vi "Receiver UI.vi"(11 "Error In":errorcluster) -> (15 "Error Out":errorcluster)   [LabVIEW 2022 SP3, in "Receiver.lvclass"]
doc: "This VI acts as a receiver and displays the data received to user."
uses:
  Receiver.lvclass
  Controls/Operation.ctl
  Controls/State Cluster.ctl
  Controls/User Event Operation.ctl
  Controls/Receiver Data Cluster.ctl
  Downloads/Sample PC Template/Sample PC Template/Typedefs/Data.ctl
  Downloads/Sample PC Template/Sample PC Template/Sample PC Template.lvlib
  Data/Data.lvclass
panel:
  out "Receiver Notified":bool
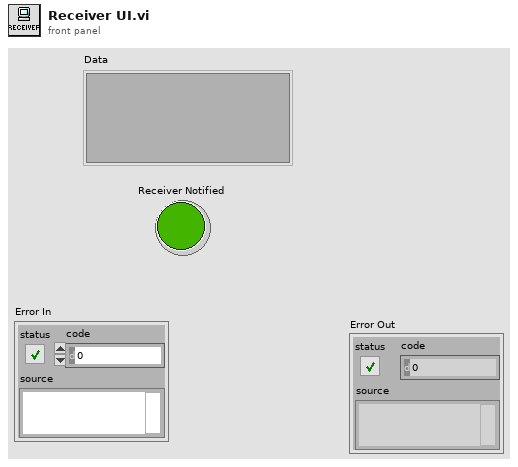
[diagram p1: front panel]
types:
  T1 = typedef "User Event Operation.ctl" = enum16{"Obtain", "Generate", "Release"}
  T2 = typedef "Receiver Data Cluster.ctl" = cluster{"Data":variant, "Receiver UI Triggered":bool, "Data.lvclass":refnum<class "Data.lvclass">, "VI Refnum":refnum<vi>}
  T3 = typedef "State Cluster.ctl" = cluster{"State":string, "Data":variant}
  T4 = typedef "Operation.ctl" = enum16{"Create", "Enqueue", "Enqueue N", "Enstack", "Dequeue", "Flush", "Release"}
  T5 = typedef "Sample PC Template.lvlib/Data.ctl" = cluster{"State":string, "Data":variant}
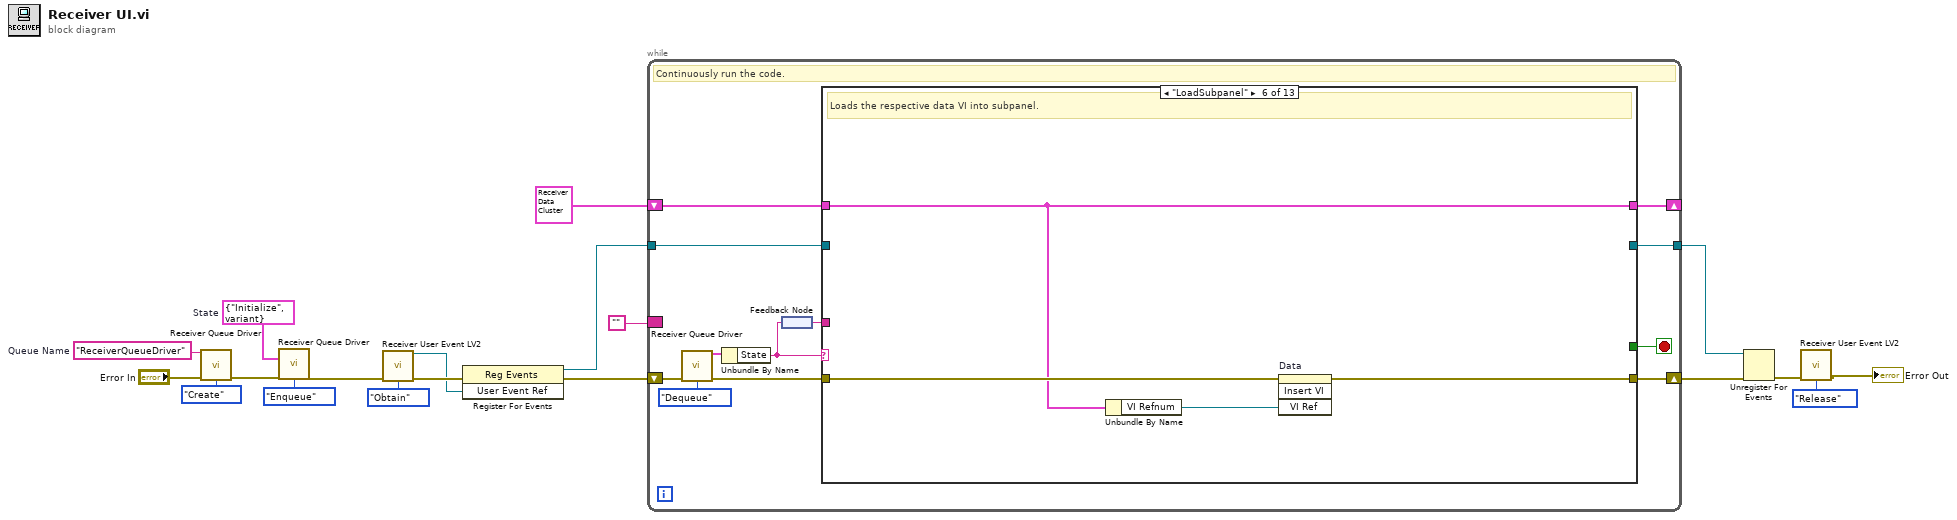
[diagram p0: block diagram]
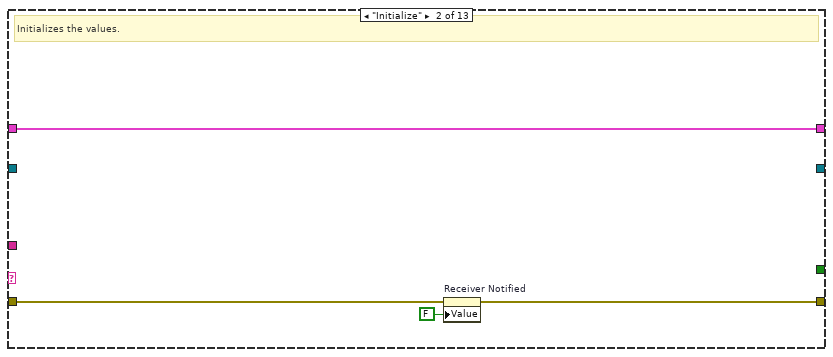
[diagram p3: hidden frame]
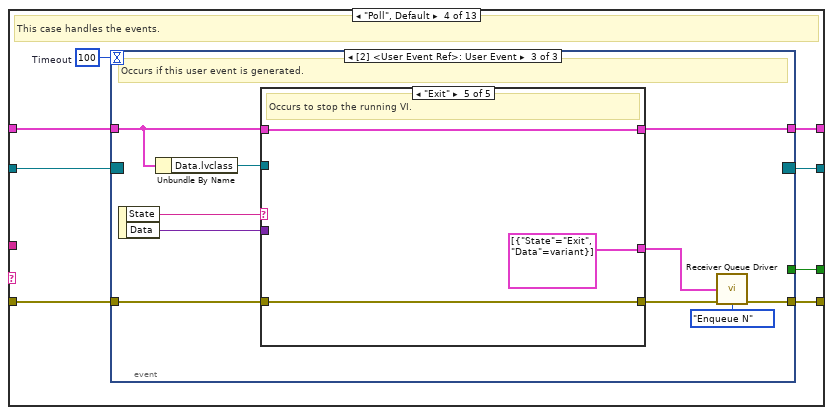
[diagram p5: hidden frame]
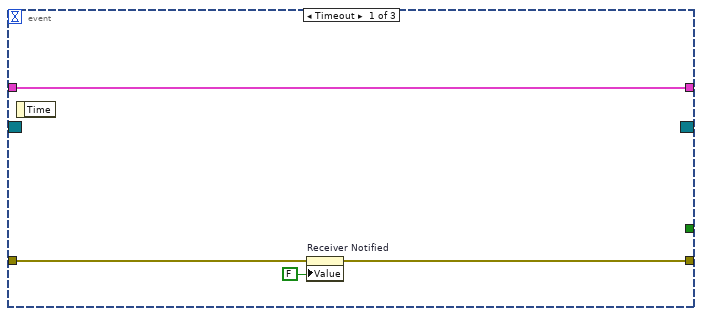
[diagram p6: hidden frame]
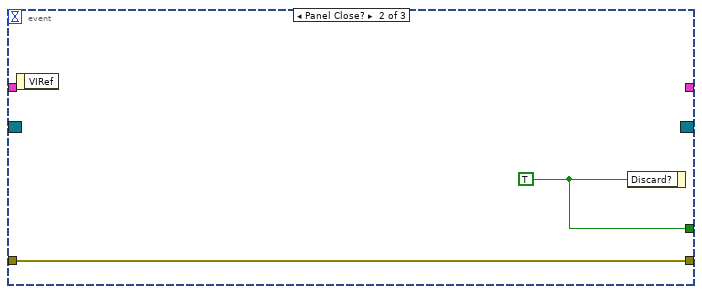
[diagram p7: hidden frame]
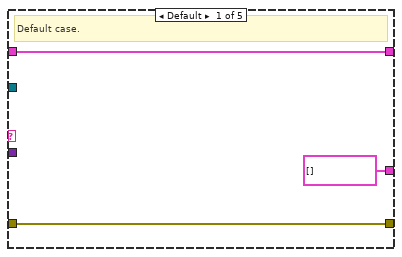
[diagram p8: hidden frame]
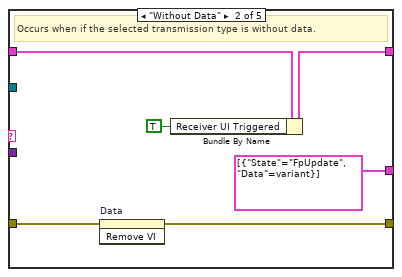
[diagram p9: hidden frame]
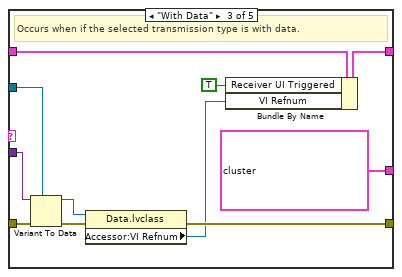
[diagram p10: hidden frame]
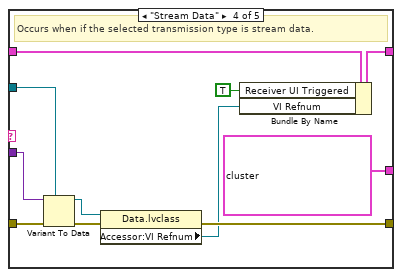
[diagram p11: hidden frame]
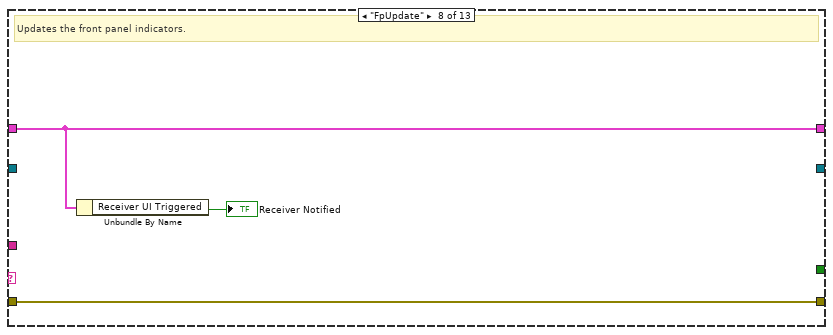
[diagram p14: hidden frame]
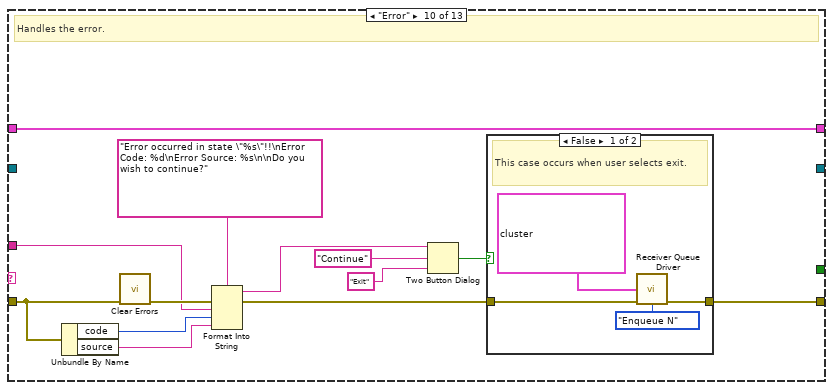
[diagram p16: hidden frame]
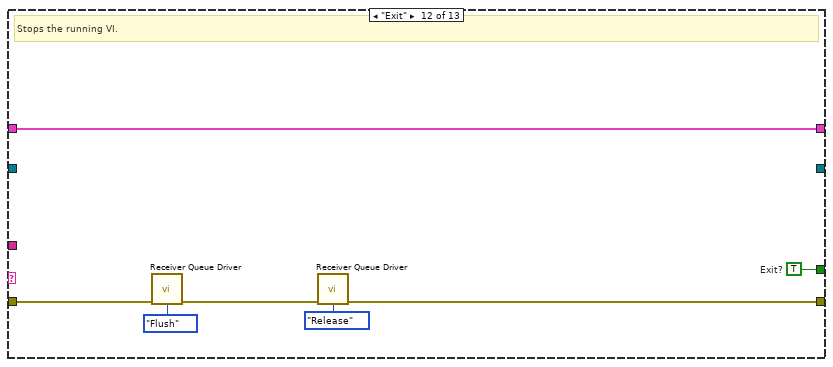
[diagram p19: hidden frame]
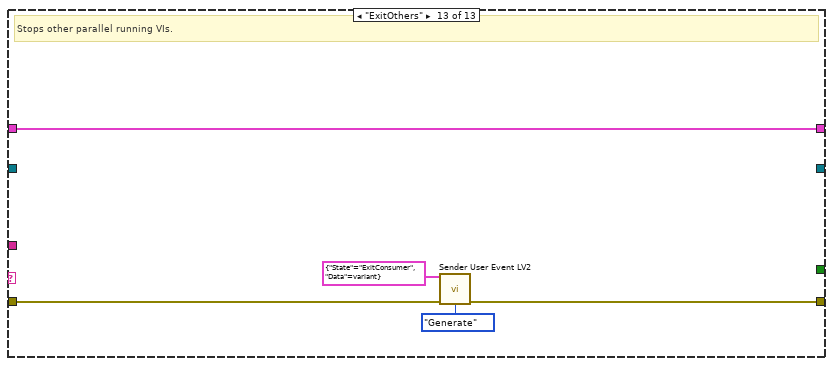
[diagram p20: hidden frame]
diagram:
  w14 = T3 {"State"="Initialize", "Data"=variant}  # State
  w15 = "ReceiverQueueDriver"  # Queue Name
  n1 = call "Receiver Queue Driver.vi"("Queue Name"=w15, "Error In"="Error In", "Operations"=Operation."Create") -> ("Error Out"=w18:errorcluster)  [unwired: 11 in, 1 out]
  n2 = call "Receiver Queue Driver.vi"("State"=w14, "Error In"=w18, "Operations"=Operation."Enqueue") -> ("Error Out"=w12:errorcluster)  [unwired: 11 in, 1 out]
  n3 = call "Receiver User Event LV2.vi"("Error In"=w12, "Operation"=User_Event_Operation."Obtain") -> ("User Event Ref"=w8:refnum<user-event>, "Error Out"=w11:errorcluster)  [unwired: 12 in]
  n4 = register-events(error in=w11, w8) -> (reference out=w7:refnum<event-registration>, error out=w9:errorcluster)  [unwired: 1 in]
  n5 = while {
    border: "" -> [_]
    shift-right: [w25] -> w5
    shift-left: w9 -> [w30]
    tunnel: w7 -> [w23]
    shift-right: [w21] -> _
    shift-left: T2 {"Data"=variant, "Receiver UI Triggered"=FALSE, "Data.lvclass"=refnum, "VI Refnum"=refnum} -> [w22]
    tunnel: [w20] -> w4
    stop <- w24 stop-if-true
    # "Continuously run the code."
    n6 = call "Receiver Queue Driver.vi"("Error In"=w30, "Operations"=Operation."Dequeue") -> ("Dequeued Element"=w29:T3, "Error Out"=w28:errorcluster)  [unwired: 12 in]
    n7 = Unbundle By Name(w29) -> ("State"=w27:string)
    n8 = feedback-in #1(w27) -> ()
    n9 = feedback #1() -> (w26:string)
    n10 = case shown="\"LoadSubpanel\"" w27 {
      tunnel: w28 -> [w33 w36 w39 w47 w99 w103 w105 w108 w110 w115 w130 w137 w142]
      tunnel: w26 -> [_ _ _ _ _ _ _ _ _ w112 _ _ _]
      tunnel: [w33 w34 w39 w45 w99 w102 w105 w108 w110 w116 w130 w134 w141] -> w25
      tunnel: [_ _ _ w44 _ _ _ _ _ _ _ w132 _] -> w24
      tunnel: w23 -> [_ _ _ w43 _ _ _ _ _ _ _ _ _]
      tunnel: w22 -> [w32 w37 w38 w42 w98 w100 w104 w107 w109 w111 w129 w131 w138]
      tunnel: [w32 w37 w38 w41 w98 w100 w104 w107 w109 w111 w129 w131 w138] -> w21
      tunnel: [_ _ _ w40 _ _ _ _ _ _ _ _ _] -> w20
      frame "/********* Initialize *********/" {
      }
      frame "Initialize" {
        # "Initializes the values."
        n11 = property on="Receiver Notified" class="Bool (strict)"(error in=w36, "Value"=FALSE ("Receiver UI Trigered")) -> (error out=w34:errorcluster)  [unwired: 1 in, 1 out]
      }
      frame "/******* Poll *********/" {
      }
      frame "Poll", Default {
        w46 = 100  # Timeout
        # "This case handles the events."
        n12 = event shown="[2] <User Event Ref>: User Event" {
          selector: w43 -> [_ _ _]
          dyn-events: [_ _ _] -> w40
          timeout: w46 -> [_ _ _]
          tunnel: w47 -> [w50 w53 w59]
          tunnel: [w49 w53 w62] -> w45
          tunnel: [_ w52 _] -> w44
          tunnel: w42 -> [w51 _ w57]
          tunnel: [w51 _ w63] -> w41
          event Timeout {
            n13 = event-data() -> ()  [unwired: 1 in, 1 out]
            n14 = property on="Receiver Notified" class="Bool (strict)"(error in=w50, "Value"=FALSE ("Receiver UI Trigered")) -> (error out=w49:errorcluster)  [unwired: 1 in, 1 out]
          }
          event Panel Close? {
            w52 = TRUE ("Discard?")
            n15 = event-data() -> ()  [unwired: 1 in, 1 out]
            n16 = event-data("Discard?"=w52) -> ()  [unwired: 1 in, 1 out]
          }
          event User Event {
            # "Occurs if this user event is generated."
            n17 = event-data() -> ("State"=w60:string, "Data"=w54:variant)  [unwired: 1 in]
            n18 = Unbundle By Name(w57) -> ("Data.lvclass"=w55:refnum<class "Data.lvclass">)
            n19 = case shown="\"Exit\"" w60 {
              tunnel: w57 -> [w65 w72 w83 w94 w97]
              tunnel: [w65 w71 w82 w93 w97] -> w63
              tunnel: w59 -> [w66 w68 w80 w91 w96]
              tunnel: [w66 w67 w79 w90 w96] -> w58
              tunnel: [T3[] [] ("State []") T3[] [{"State"="FpUpdate", "Data"=variant}] ("State []") T3[] [{"State"="LoadSubpanel", "Data"=variant}, {"State"="FpUpdate", "Data"=variant}] ("State []") T3[] [{"State"="LoadSubpanel", "Data"=variant}, {"State"="FpUpdate", "Data"=variant}] ("State []") T3[] [{"State"="Exit", "Data"=variant}] ("State []")] -> w56
              tunnel: w55 -> [_ _ w74 w85 _]
              tunnel: w54 -> [_ _ w75 w86 _]
              frame Default {
                # "Default case."
              }
              frame "Without Data" {
                # "Occurs when if the selected transmission type is without data."
                n20 = invoke on="Data" class="SubPnl" method="Remove VI"(error in=w68) -> (error out=w67:errorcluster)  [unwired: 2 in, 2 out]
                n21 = Bundle By Name(cluster=w72, "Receiver UI Triggered"=TRUE) -> (w71:T2)
              }
              frame "With Data" {
                # "Occurs when if the selected transmission type is with data."
                n22 = Variant To Data(error in=w80, type=w74, Variant=w75) -> (data=w73:refnum<class "Data.lvclass">, error out=w76:errorcluster)
                n23 = property class="Data.lvclass"(reference=w73, error in=w76) -> (error out=w79:errorcluster, "Accessor:VI Refnum"=w78:refnum<vi>)  [unwired: 1 out]
                n24 = Bundle By Name(cluster=w83, "Receiver UI Triggered"=TRUE, "VI Refnum"=w78) -> (w82:T2)
              }
              frame "Stream Data" {
                # "Occurs when if the selected transmission type is stream data."
                n25 = Variant To Data(error in=w91, type=w85, Variant=w86) -> (data=w84:refnum<class "Data.lvclass">, error out=w87:errorcluster)
                n26 = property class="Data.lvclass"(reference=w84, error in=w87) -> (error out=w90:errorcluster, "Accessor:VI Refnum"=w89:refnum<vi>)  [unwired: 1 out]
                n27 = Bundle By Name(cluster=w94, "Receiver UI Triggered"=TRUE, "VI Refnum"=w89) -> (w93:T2)
              }
              frame "Exit" {
                # "Occurs to stop the running VI."
              }
            }
            n28 = call "Receiver Queue Driver.vi"("State []"=w56, "Error In"=w58, "Operations"=Operation."Enqueue N") -> ("Error Out"=w62:errorcluster)  [unwired: 11 in, 1 out]
          }
        }
      }
      frame "/******* Functionality *********/" {
      }
      frame "LoadSubpanel" {
        # "Loads the respective data VI into subpanel."
        n29 = Unbundle By Name(w100) -> ("VI Refnum"=w101:refnum<vi>)
        n30 = invoke on="Data" class="SubPnl" method="Insert VI"(error in=w103, "VI Ref"=w101) -> (error out=w102:errorcluster)  [unwired: 2 in, 3 out]
      }
      frame "/********* Front panel updates ********/" {
      }
      frame "FpUpdate" {
        # "Updates the front panel indicators."
        n31 = Unbundle By Name(w107) -> ("Receiver UI Triggered"=→"Receiver Notified":bool)
      }
      frame "/******** Error Handling ********/" {
      }
      frame "Error" {
        # "Handles the error."
        n32 = Unbundle By Name(w115) -> ("code"=w113:i32, "source"=w114:string)
        n33 = call <vilib>:"Clear Errors.vi"("error in (no error)"=w115) -> ("error out"=w123:errorcluster)  [unwired: 5 in, 1 out]
        n34 = Format Into String(format string="Error occurred in state \"%s\"!!\nError Code: %d\nError Source: %s\n\nDo you wish to continue?", error in=w123, w112, w113, w114) -> (resulting string=w121:string, error out=w118:errorcluster)  [unwired: 1 in]
        n35 = Two Button Dialog(message=w121, 1:"Exit" ("F button name (\"Cancel\")"), 2:"Continue" ("T button name (\"OK\")")) -> (T button?=w117:bool)
        n36 = case shown="False" w117 {
          tunnel: w118 -> [w127 w128]
          tunnel: [w126 w128] -> w116
          frame False {
            # "This case occurs when user selects exit."
            n37 = call "Receiver Queue Driver.vi"("State []"=T3[] [{"State"="ExitOthers", "Data"=variant}, {"State"="Exit", "Data"=variant}], "Error In"=w127, "Operations"=Operation."Enqueue N") -> ("Error Out"=w126:errorcluster)  [unwired: 11 in, 1 out]
          }
          frame True {
            # "This case occurs when user selects to continue."
          }
        }
      }
      frame "/******* Exit *********/" {
      }
      frame "Exit" {
        w132 = TRUE  # Exit?
        # "Stops the running VI."
        n38 = call "Receiver Queue Driver.vi"("Error In"=w137, "Operations"=Operation."Flush") -> ("Error Out"=w135:errorcluster)  [unwired: 12 in, 1 out]
        n39 = call "Receiver Queue Driver.vi"("Error In"=w135, "Operations"=Operation."Release") -> ("Error Out"=w134:errorcluster)  [unwired: 12 in, 1 out]
      }
      frame "ExitOthers" {
        # "Stops other parallel running VIs."
        n40 = call "Sender User Event LV2.vi"("Data"=T5 {"State"="ExitConsumer", "Data"=variant}, "Error In"=w142, "Operation"=User_Event_Operation."Generate") -> ("Error Out"=w141:errorcluster)  [unwired: 11 in, 1 out]
      }
    }
  }
  n41 = Unregister For Events(event registration refnum=w4, error in=w5) -> (error out=w3:errorcluster)
  n42 = call "Receiver User Event LV2.vi"("Error In"=w3, "Operation"=User_Event_Operation."Release") -> ("Error Out"=→"Error Out":errorcluster)  [unwired: 12 in, 1 out]
